vi "Write Deviate.vi"(8 "error in (no error)":errorcluster, 10 "Deviate":bool, 11 "Path Settings in":refnum<class "Path Settings.lvclass">) -> (0 "error out":errorcluster, 3 "Path Settings out":refnum<class "Path Settings.lvclass">)   [LabVIEW 2019, in "Path Settings.lvclass"]
uses:
  Path Settings.lvclass
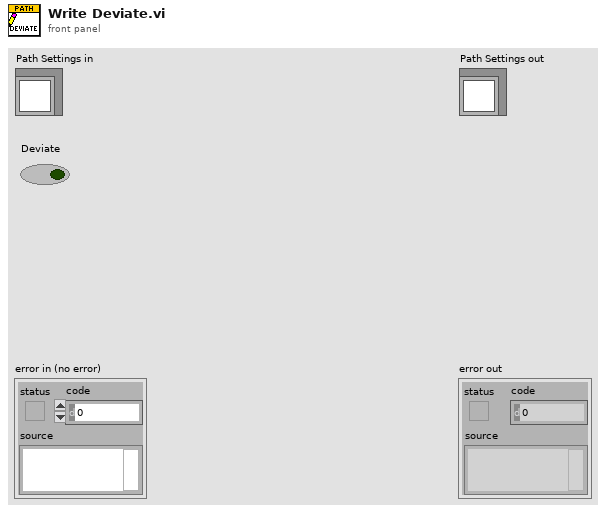
[diagram p1: front panel]
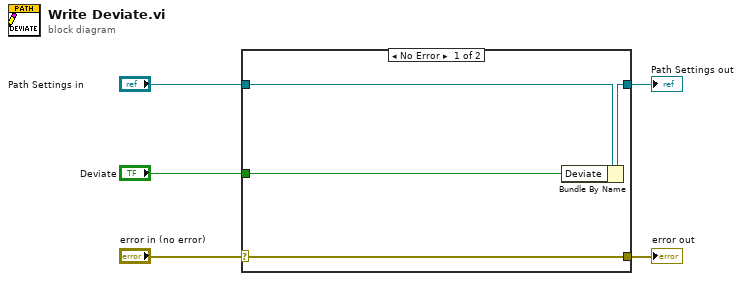
[diagram p0: block diagram]
diagram:
  n1 = case shown="No Error" "error in (no error)" {
    selector: "error in (no error)" -> [w9 w10]
    tunnel: [w9 w10] -> w4
    tunnel: [w7 w11] -> w2
    tunnel: "Path Settings in" -> [w8 w11]
    tunnel: "Deviate" -> [w6 _]
    frame No Error {
      n2 = Bundle By Name(cluster=w8, "Deviate"=w6) -> (w7:refnum<class "Path Settings.lvclass">)
    }
    frame Error {
    }
  }
  "error out" <- w4
  "Path Settings out" <- w2
